vi "UDP Send and Receive (repeat on error).vi"(6 "Number of retries (3)":u8=3, 7 "timeout ms (100)":i32=100, 8 "error in (no error)":errorcluster, 9 "Data":string, 10 "IP":string, 11 "connection ID in":refnum<k16>) -> (0 "error out":errorcluster, 1 "Received Data":T1, 2 "ACK/NACK":T2, 3 "connection ID out":refnum<k16>)   [LabVIEW 2016, in "SMD-7615.lvlib" / "eSCL.lvlib"]
doc: "This is the core of UDP send and receive. If a UDP communication timeout is detected VI retries for a given umber of times.\nVI returns an Error if UDP communciation error exceeded number of trials. \nVI returns an Error if Input Parameter \"Number of retries\" N is not within ( 1 <= N < 10)"
uses:
  eSCL.lvlib
  UDP ACK NACK.ctl
  UDP Received Data.ctl
  <vilib>/GPower/Error/Library/ErrorType.vi
  <vilib>/GPower/Error/Library/SplitAppended.vi
  <vilib>/GPower/Error/Library/SubVIs/ExplanationToError.vi
  <vilib>/dlg_ctls.llb/Space Constant.vi
  <vilib>/Utility/error.llb/Trim Whitespace.vi
  <vilib>/Utility/error.llb/Error Code Database.vi
  <vilib>/GPower/Error/Library/SubVIs/SetStatus.vi
  <vilib>/GPower/Error/Library/Append/AppendSingle.vi
  <vilib>/GPower/Error/GPError.lvlib
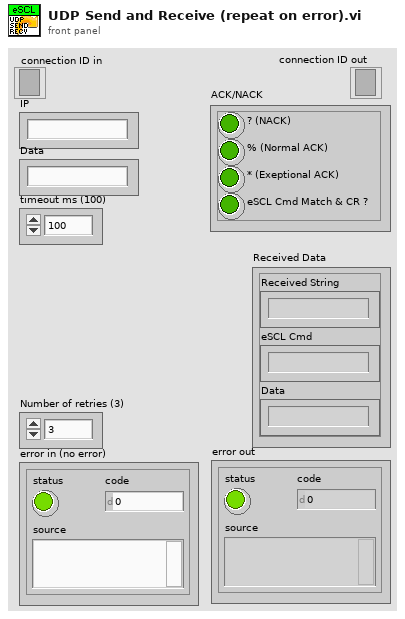
[diagram p1: front panel]
types:
  T1 = typedef "SMD-7615.lvlib/eSCL.lvlib/UDP Received Data.ctl" = cluster{"Received String":string, "eSCL Cmd":string, "Data":string}
  T2 = typedef "SMD-7615.lvlib/eSCL.lvlib/UDP ACK NACK.ctl" = cluster{"? (NACK)":bool, "% (Normal ACK)":bool, "* (Exeptional ACK)":bool, "eSCL Cmd Match & CR ?":bool}
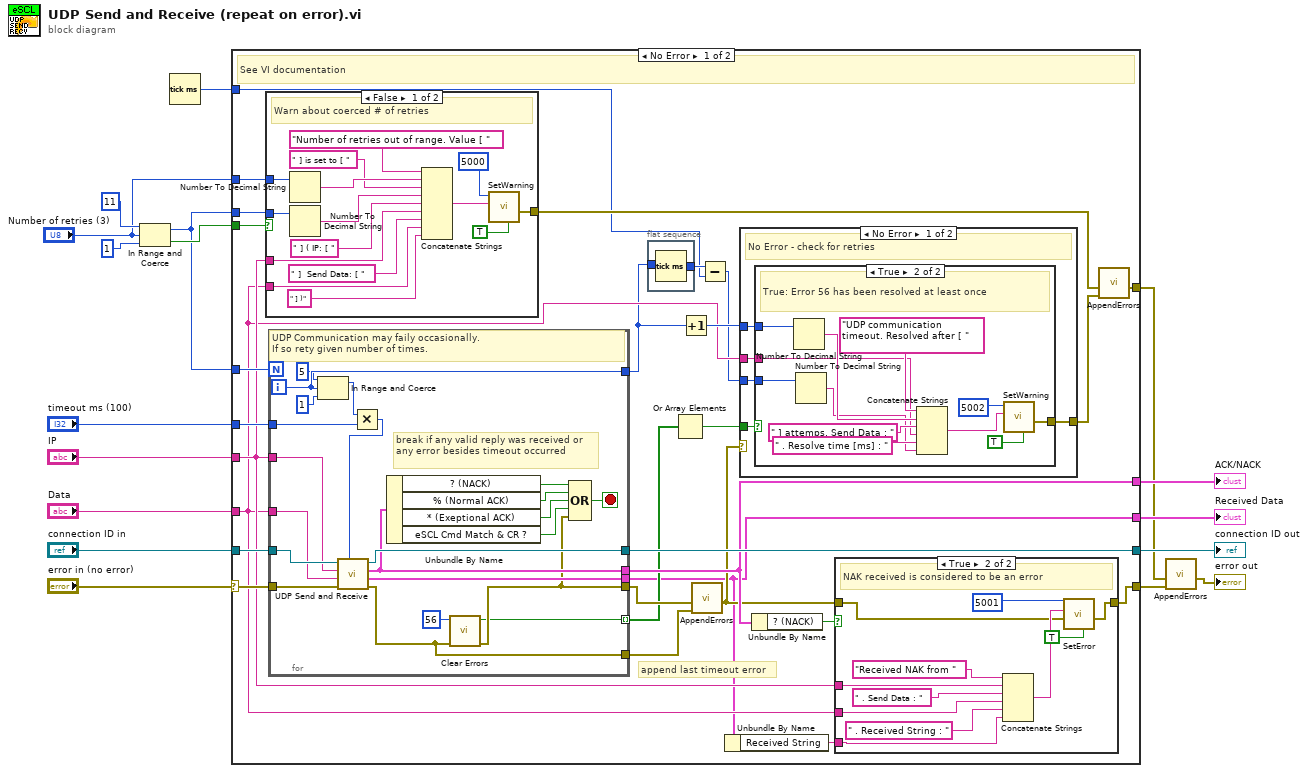
[diagram p0: block diagram]
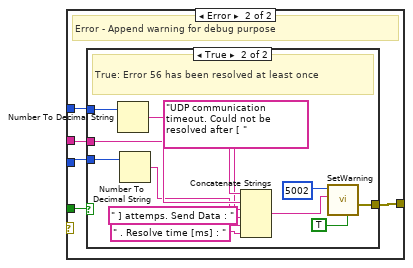
[diagram p3: hidden frame]
diagram:
  n1 = In Range and Coerce(upper limit=u8 11, x="Number of retries (3)", lower limit=u8 1) -> (coerced(x)=w4:u8, In Range?=w5:bool)
  n2 = Tick Count (ms)() -> (millisecond timer value=w1:u32)
  n3 = case shown="No Error" "error in (no error)" {
    selector: "error in (no error)" -> [w45 w130]
    tunnel: "connection ID in" -> [w44 w131]
    tunnel: [w42 w131] -> w15
    tunnel: [w38 w130] -> w9
    tunnel: "timeout ms (100)" -> [w43 _]
    tunnel: "IP" -> [w30 _]
    tunnel: "Data" -> [w24 _]
    tunnel: [w19 _] -> w13
    tunnel: [w37 _] -> w12
    tunnel: w4 -> [w41 _]
    tunnel: w5 -> [w35 _]
    tunnel: w4 -> [w34 _]
    tunnel: "Number of retries (3)" -> [w33 _]
    tunnel: [w26 _] -> w2
    tunnel: w1 -> [w21 _]
    frame No Error {
      # "append last timeout error"
      # "See VI documentation"
      n4 = case shown="False" w35 {
        tunnel: [w95 _] -> w28
        tunnel: w30 -> [w87 _]
        tunnel: w24 -> [w85 _]
        tunnel: w33 -> [w83 _]
        tunnel: w34 -> [w82 _]
        frame False {
          # "Warn about coerced # of retries"
          n5 = Number To Decimal String(number=w83) -> (decimal integer string=w93:string)  [unwired: 1 in]
          n6 = Number To Decimal String(number=w82) -> (decimal integer string=w90:string)  [unwired: 1 in]
          n7 = Concatenate Strings("Number of retries out of range. Value [ " ("string"), w93, " ] is set to [ " ("string"), w90, " ] ( IP: [ " ("string"), w87, " ]  Send Data: [ " ("string"), w85, " ] )" ("string")) -> (w89:string)
          n8 = call <vilib>:"SetWarning.vi"("Append timestamp?"=TRUE, "Warning description"=w89, "Warning code"=5000) -> ("Error out"=w95:errorcluster)  [unwired: 8 in]
        }
        frame True {
          # "# of retries within limits - no warning"
        }
      }
      n9 = for {
        N: w41 -> [_]
        tunnel: w43 -> [w109]
        tunnel: w30 -> [w127]
        tunnel: w24 -> [w126]
        tunnel: [w124] -> w19
        tunnel: [w123] -> w37
        tunnel: [w116] -> w39
        tunnel: [w114] -> w32 mode=indexing
        tunnel: [w112] -> w23
        tunnel: w45 -> [w129]
        tunnel: [w117] -> w40
        tunnel: w44 -> [w128]
        tunnel: [w125] -> w42
        i -> [w112]
        stop <- w118 stop-if-true
        # "break if any valid reply was received or any error besides timeout occurred"
        # "UDP Communication may faily occasionally. \nIf so rety given number of times."
        n10 = In Range and Coerce(upper limit=5, x=w112, lower limit=1) -> (coerced(x)=w113:i32)  [unwired: 1 out]
        n11 = Multiply(x=w113, y=w109) -> (x*y=w108:i32)
        n12 = call "UDP Send and Receive.vi"("timeout ms (100)"=w108, "error in (no error)"=w129, "Data"=w126, "IP"=w127, "connection ID in"=w128) -> ("error out"=w116:errorcluster, "Received Data"=w124:T1, "ACK/NACK"=w123:T2, "connection ID out"=w125:refnum<k16>)  [unwired: 3 in]
        n13 = Unbundle By Name(w123) -> ("? (NACK)"=w122:bool, "% (Normal ACK)"=w121:bool, "* (Exeptional ACK)"=w120:bool, "eSCL Cmd Match & CR ?"=w119:bool)
        n14 = call <vilib>:"Clear Errors.vi"("error in (no error)"=w116, "specific error code to clear (0: all)"=56) -> ("error out"=w117:errorcluster, "specific error cleared?"=w114:bool)  [unwired: 4 in]
        n15 = Compound Arithmetic op=OR(w122, w121, w120, w119, w117) -> (w118:bool)
      }
      n16 = flat-sequence {
        tunnel: w23 -> [_]
        tunnel: [w46] -> w22
        frame #0 {
          n17 = Tick Count (ms)() -> (millisecond timer value=w46:u32)
        }
      }
      n18 = Or Array Elements(Boolean array=w32) -> (logical OR=w31:bool)
      n19 = Increment(x=w23) -> (x+1=w25:i32)
      n20 = call-poly <vilib>:"AppendErrors.vi"("Error to append"=w39, "Error in"=w40) -> ("Appended errors out"=w29:errorcluster)  [unwired: 9 in]
      n21 = Subtract(x=w22, y=w21) -> (x-y=w20:u32)
      n22 = Unbundle By Name(w19) -> ("Received String"=w18:string)
      n23 = case shown="No Error" w29 {
        tunnel: w31 -> [w51 w66]
        tunnel: w25 -> [w50 w68]
        tunnel: [w49 w65] -> w27
        tunnel: w24 -> [w48 w67]
        tunnel: w20 -> [w47 w64]
        frame No Error {
          # "No Error - check for retries"
          n24 = case shown="True" w51 {
            tunnel: [_ w63] -> w49
            tunnel: w50 -> [_ w61]
            tunnel: w48 -> [_ w55]
            tunnel: w47 -> [_ w54]
            frame False {
              # "False: No Error, No Warning"
            }
            frame True {
              # "True: Error 56 has been resolved at least once"
              n25 = Number To Decimal String(number=w61) -> (decimal integer string=w58:string)  [unwired: 1 in]
              n26 = Number To Decimal String(number=w54) -> (decimal integer string=w52:string)  [unwired: 1 in]
              n27 = Concatenate Strings("UDP communication timeout. Resolved after [ " ("string"), w58, " ] attemps. Send Data : " ("string"), w55, " . Resolve time [ms] : " ("string"), w52) -> (w57:string)
              n28 = call <vilib>:"SetWarning.vi"("Append timestamp?"=TRUE, "Warning description"=w57, "Warning code"=5002 ("Error code")) -> ("Error out"=w63:errorcluster)  [unwired: 8 in]
            }
          }
        }
        frame Error {
          # "Error - Append warning for debug purpose"
          n29 = case shown="True" w66 {
            tunnel: [_ w80] -> w65
            tunnel: w68 -> [_ w78]
            tunnel: w67 -> [_ w72]
            tunnel: w64 -> [_ w71]
            frame False {
              # "False: No Error, No Warning"
            }
            frame True {
              # "True: Error 56 has been resolved at least once"
              n30 = Number To Decimal String(number=w78) -> (decimal integer string=w75:string)  [unwired: 1 in]
              n31 = Number To Decimal String(number=w71) -> (decimal integer string=w69:string)  [unwired: 1 in]
              n32 = Concatenate Strings("UDP communication timeout. Could not be resolved after [ " ("string"), w75, " ] attemps. Send Data : " ("string"), w72, " . Resolve time [ms] : " ("string"), w69) -> (w74:string)
              n33 = call <vilib>:"SetWarning.vi"("Append timestamp?"=TRUE, "Warning description"=w74, "Warning code"=5002 ("Error code")) -> ("Error out"=w80:errorcluster)  [unwired: 8 in]
            }
          }
        }
      }
      n34 = Unbundle By Name(w37) -> ("? (NACK)"=w36:bool)
      n35 = case shown="True" w36 {
        tunnel: w29 -> [w96 w100]
        tunnel: [w96 w103] -> w38
        tunnel: w30 -> [_ w105]
        tunnel: w24 -> [_ w104]
        tunnel: w18 -> [_ w97]
        frame False {
        }
        frame True {
          # "NAK received is considered to be an error"
          n36 = Concatenate Strings("Received NAK from " ("string"), w105, " . Send Data : " ("string"), w104, " . Received String : " ("string"), w97) -> (w102:string)
          n37 = call <vilib>:"SetError.vi"("Append timestamp?"=TRUE, "Error in"=w100, "Error description"=w102, "Error code"=5001) -> ("Error out"=w103:errorcluster)  [unwired: 7 in]
        }
      }
      n38 = call-poly <vilib>:"AppendErrors.vi"("Error to append"=w27, "Error in"=w28) -> ("Appended errors out"=w26:errorcluster)  [unwired: 9 in]
    }
    frame Error {
    }
  }
  "connection ID out" <- w15
  "ACK/NACK" <- w12
  "Received Data" <- w13
  n39 = call-poly <vilib>:"AppendErrors.vi"("Error to append"=w9, "Error in"=w2) -> ("Appended errors out"=→"error out":errorcluster)  [unwired: 9 in]
